vi "update_parameters.vi"(0 "Modify":T1, 9 "Parameters":T2={"Stimulus"={"Type"=enum."Off", "Phase"=0.0, "Amplitude"=[], "Injection point"=enum."Total pose", "Closed loop"=FALSE, "Offset"=[], "Tip -> world"=FALSE, "Frequency"=0.0, "Length"=0.0}, "Goal Filter A"={"Speedup max"=0.0, "Speedup thresh"=0.0, "Speedup nonlin"=0.0, "Filters"=[]}, "Mode controls"={"Hold"=FALSE, "Cancellation"=FALSE, "Goal filter"=FALSE, "Trigger"=FALSE}, "Manipulator type"=enum."Current piezo", "Manipulator calibration"={"Tool offsets"=[[0.0, 0.0, 36200.0]], "Handle light calibration"=[], "Base pivots"=[], "Output pivots"=[], "Length center"=0.0, "Workspace height"=[], "Workspace diameter"=[0.0, 0.0, 36200.0], "Stack travel"=400.0, "Saturation pos"=375.0, "Inverse filters"=[], "Strut length"=0.0}, "Network"={"Remote Host"="", "Send Status"=FALSE, "Send Port"=0, "Recv Commands"=FALSE, "Recv Port"=0}, "Goal Filter B"={"Speedup max"=0.0, "Speedup thresh"=0.0, "Speedup nonlin"=0.0, "Filters"=[]}, "Cancellation"={"KP"={"XY"=0.0, "Rxy"=0.0, "Z"=0.0, "Rz"=0.0}, "KI"=0.0, "KD"={"XY"=0.0, "Rxy"=0.0, "Z"=0.0, "Rz"=0.0}, "Max vel"=20.0, "Max acc"=0.001, "Int error limit"=3.0, "RCM gain"=0.0, "Bypass"=FALSE, "Degraded gain"=0.0}, "Transition time"=0.0, "Estimation"={"Link"={"Measure noise"=[], "Process noise"=[], "Alt process noise"=[], "Alt turnoff cycles"=20, "Innovation limit"=[], "Residue threshold"=0.0, "Enable"=FALSE}, "Handle"={"Measure noise"=[], "Process noise"=[], "State limits"=[], "Innovation limit"=[], "Prediction Lookahead"=0.0, "Enable"=FALSE}}} {"Transition time" format="%_3f"; "Cancellation"."Degraded gain" min=0 max=1 step=0.1 format="%#_3p"; "Cancellation"."RCM gain" min=0 max=1 step=0.1 format="%#_3p"; "Cancellation"."KD"."Rz" min=-1 max=1 step=0.01 format="%#_3p"; "Cancellation"."KD"."Rxy" min=-1 max=1 step=0.01 format="%#_3p"; "Cancellation"."KD"."Z" min=-1 max=1 step=0.01 format="%#_3p"; "Cancellation"."KD"."XY" min=-1 max=1 step=0.01 format="%#_3p"; "Cancellation"."KI" min=0 max=1 step=0.01 format="%#_3p"; "Cancellation"."KP"."Rz" min=-1 max=1 step=0.01 format="%#_3p"; "Cancellation"."KP"."Rxy" min=-1 max=1 step=0.01 format="%#_3p"; "Cancellation"."KP"."Z" min=-1 max=1 step=0.01 format="%#_3p"; "Cancellation"."KP"."XY" min=-1 max=1 step=0.01 format="%#_3p"; "Cancellation"."Max acc" format="%#_3p"; "Goal Filter B"."Filters"."V limit range" format="%_3p"; "Goal Filter B"."Filters"."V limit" format="%_3p"; "Goal Filter B"."Filters"."Upper Q" format="%_3f"; "Goal Filter B"."Filters"."Upper Fc" format="%_3p"; "Goal Filter B"."Filters"."Lower Q" format="%_3f"; "Goal Filter B"."Filters"."Scale factor" format="%_3f"; "Goal Filter B"."Filters"."Lower Fc" format="%_3p"; "Goal Filter B"."Speedup nonlin" format="%_3p"; "Goal Filter B"."Speedup thresh" format="%_3p"; "Goal Filter B"."Speedup max" format="%_3p"; "Manipulator calibration"."Strut length" format="%#_4p"; "Manipulator calibration"."Saturation pos" format="%#.1f"; "Manipulator calibration"."Stack travel" format="%#.1f"; "Manipulator calibration"."Length center" format="%#_4p"; "Manipulator calibration"."Output pivots" format="%#_6f"; "Manipulator calibration"."Base pivots" format="%#_6f"; "Manipulator calibration"."Handle light calibration" format="%#.1f"; "Goal Filter A"."Filters"."V limit range" format="%_3p"; "Goal Filter A"."Filters"."V limit" format="%_3p"; "Goal Filter A"."Filters"."Upper Q" format="%_3f"; "Goal Filter A"."Filters"."Upper Fc" format="%_3p"; "Goal Filter A"."Filters"."Lower Q" format="%_3f"; "Goal Filter A"."Filters"."Scale factor" format="%_3f"; "Goal Filter A"."Filters"."Lower Fc" format="%_3p"; "Goal Filter A"."Speedup nonlin" format="%_3p"; "Goal Filter A"."Speedup thresh" format="%_3p"; "Goal Filter A"."Speedup max" format="%_3p"; "Stimulus"."Length" min=0.0 max=100.0 step=100.0 format="%#_4p"; "Stimulus"."Frequency" min=0.0 step=100.0 format="%#_4g"; "Stimulus"."Offset" format="%#_3p"; "Stimulus"."Amplitude" format="%#_3p"; "Stimulus"."Phase" min=-180.0 max=360.0 step=100.0 format="%#.2f"}, 11 "error in":errorcluster) -> (4 "Changed":bool, 15 "error out":errorcluster)   [LabVIEW 2014]
uses:
  Micron params.ctl
  stimulus.ctl
  injection_point.ctl
  filtering/goal_loop_parms.ctl
  mode_conrols.ctl
  manipulator_cal.ctl
  asap/labview/testing/probe_calibration.ctl
  host/network_params.ctl
  cancellation/sq_control_params.ctl
  cancellation/decoupled_gain.ctl
  cancellation/estimation_controls.ctl
  ui_override_opts.ctl
  initialization/micron_globals.vi
panel:
  out "Old param string":string
  # "True if the current  parameters actually changed."
  # "Modify only these parts of the current parameters.  Other parts of the system may be in charge of other parts of the parameters.  See ui_override.vi, which generates this cluster."
  # "Locals:"
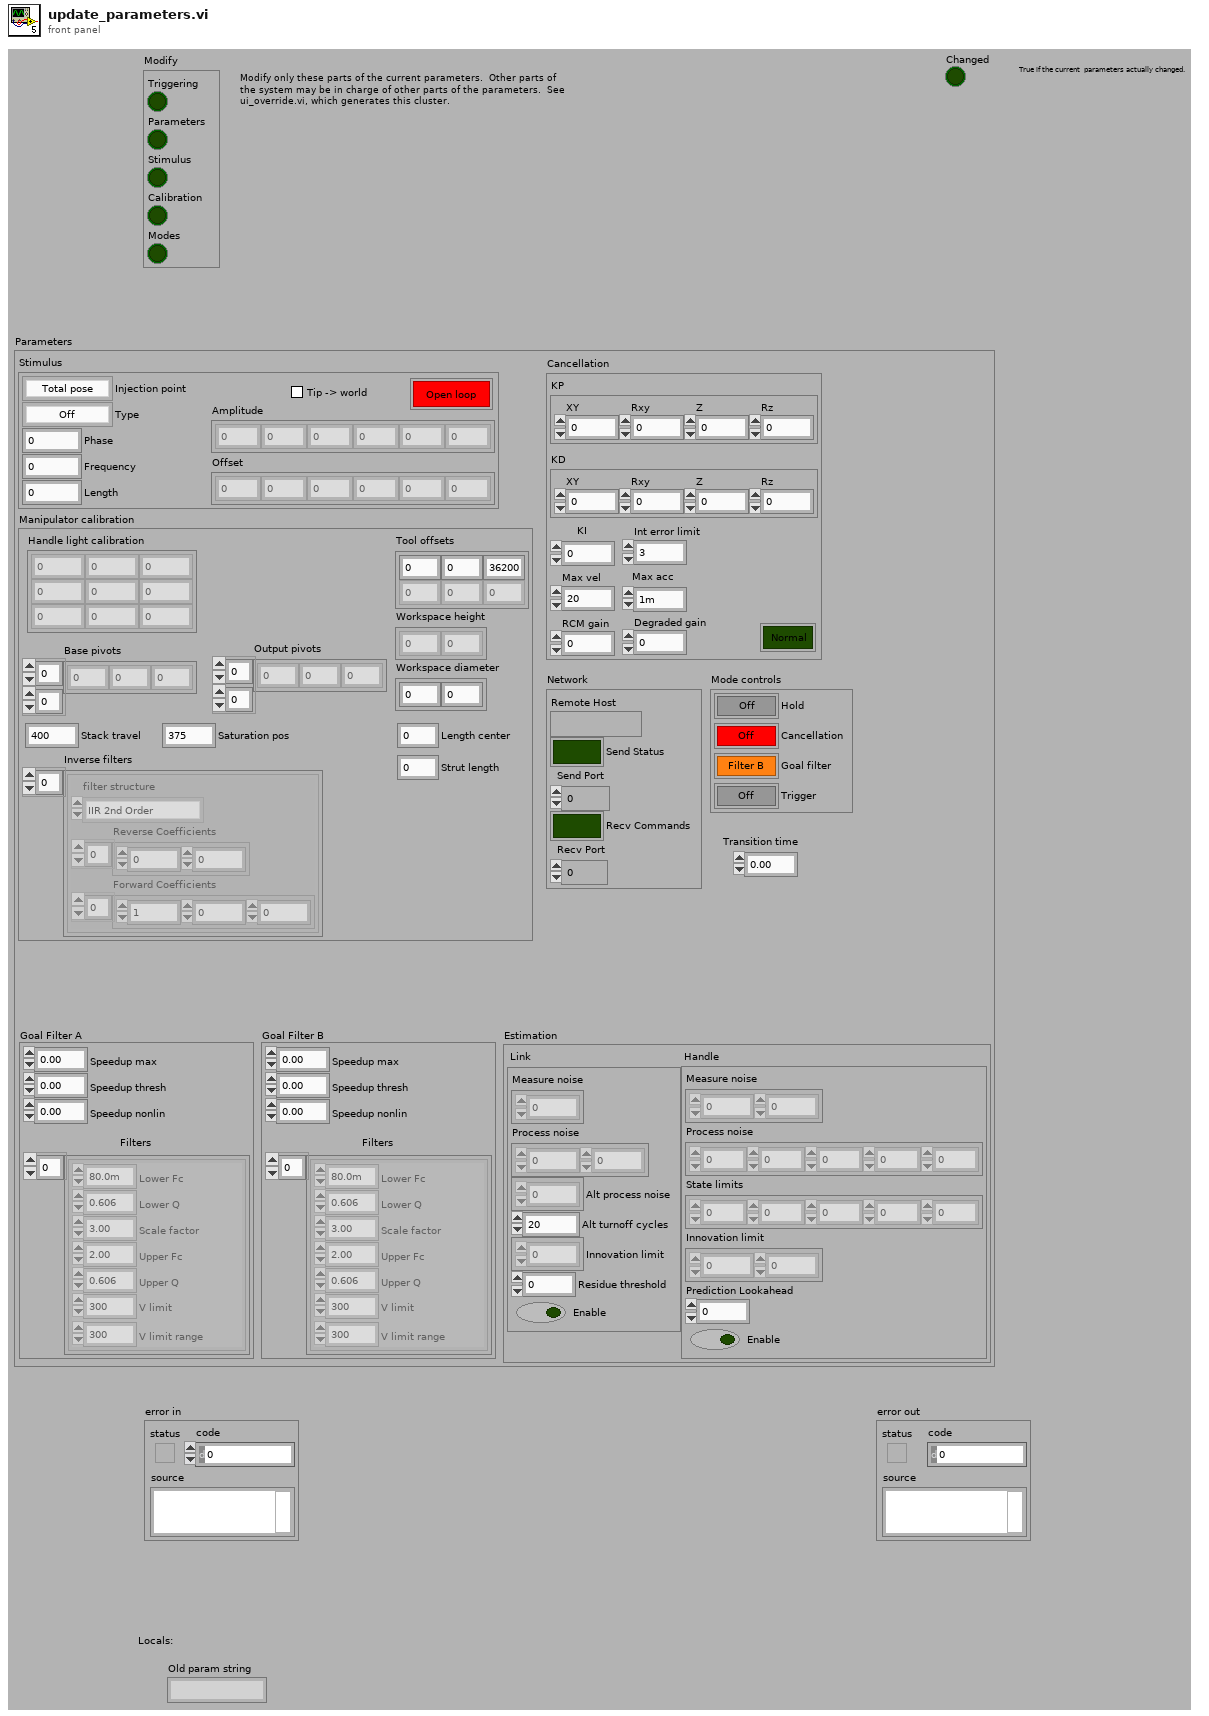
[diagram p1: front panel]
types:
  T1 = typedef "ui_override_opts.ctl" = cluster{"Triggering":bool, "Parameters":bool, "Stimulus":bool, "Calibration":bool, "Modes":bool}
  T2 = typedef "Micron params.ctl" = cluster{"Stimulus":T3, "Goal Filter A":T5, "Mode controls":T6, "Manipulator type":enum16{"Current piezo", "Voltage piezo"}, "Manipulator calibration":T7, "Network":T9, "Goal Filter B":T5, "Cancellation":T10, "Transition time":sgl, "Estimation":T12}
  T3 = typedef "stimulus.ctl" = cluster{"Type":enum16{"Off", "Step", "Sine", "Triangle", "Arbitrary"}, "Phase":dbl, "Amplitude":sgl[], "Injection point":T4, "Closed loop":bool, "Offset":sgl[], "Tip -> world":bool, "Frequency":dbl, "Length":dbl}
  T4 = typedef "injection_point.ctl" = enum16{"Total pose", "V limiter", "Goal ", "Link position", "KF link position", "Inverse kin", "Link goal", "Link error", "Controller", "Output", "Drive", "Light"}
  T5 = typedef "goal_loop_parms.ctl" = cluster{"Speedup max":sgl, "Speedup thresh":sgl, "Speedup nonlin":sgl, "Filters":cluster{"Lower Fc":sgl, "Lower Q":sgl, "Scale factor":sgl, "Upper Fc":sgl, "Upper Q":sgl, "V limit":sgl, "V limit range":sgl}[]}
  T6 = typedef "mode_conrols.ctl" = cluster{"Hold":bool, "Cancellation":bool, "Goal filter":bool, "Trigger":bool}
  T7 = typedef "manipulator_cal.ctl" = cluster{"Tool offsets":sgl[][], "Handle light calibration":T8, "Base pivots":sgl[][], "Output pivots":sgl[][], "Length center":sgl, "Workspace height":sgl[], "Workspace diameter":sgl[], "Stack travel":sgl, "Saturation pos":sgl, "Inverse filters":cluster{"filter structure":enum32{"IIR 2nd Order", "IIR 4th Order"}, "Reverse Coefficients":dbl[], "Forward Coefficients":dbl[]}[], "Strut length":sgl}
  T8 = typedef "probe_calibration.ctl" = sgl[][]
  T9 = typedef "network_params.ctl" = cluster{"Remote Host":string, "Send Status":bool, "Send Port":u16, "Recv Commands":bool, "Recv Port":u16}
  T10 = typedef "sq_control_params.ctl" = cluster{"KP":T11, "KI":sgl, "KD":T11, "Max vel":sgl, "Max acc":sgl, "Int error limit":sgl, "RCM gain":sgl, "Bypass":bool, "Degraded gain":sgl}
  T11 = typedef "decoupled_gain.ctl" = cluster{"XY":sgl, "Rxy":sgl, "Z":sgl, "Rz":sgl}
  T12 = typedef "estimation_controls.ctl" = cluster{"Link":cluster{"Measure noise":dbl[], "Process noise":dbl[], "Alt process noise":dbl[], "Alt turnoff cycles":i32, "Innovation limit":dbl[], "Residue threshold":dbl, "Enable":bool}, "Handle":cluster{"Measure noise":dbl[], "Process noise":dbl[], "State limits":dbl[], "Innovation limit":dbl[], "Prediction Lookahead":sgl, "Enable":bool}}
  T13 = enum16{"Off", "Step", "Sine", "Triangle", "Arbitrary"}
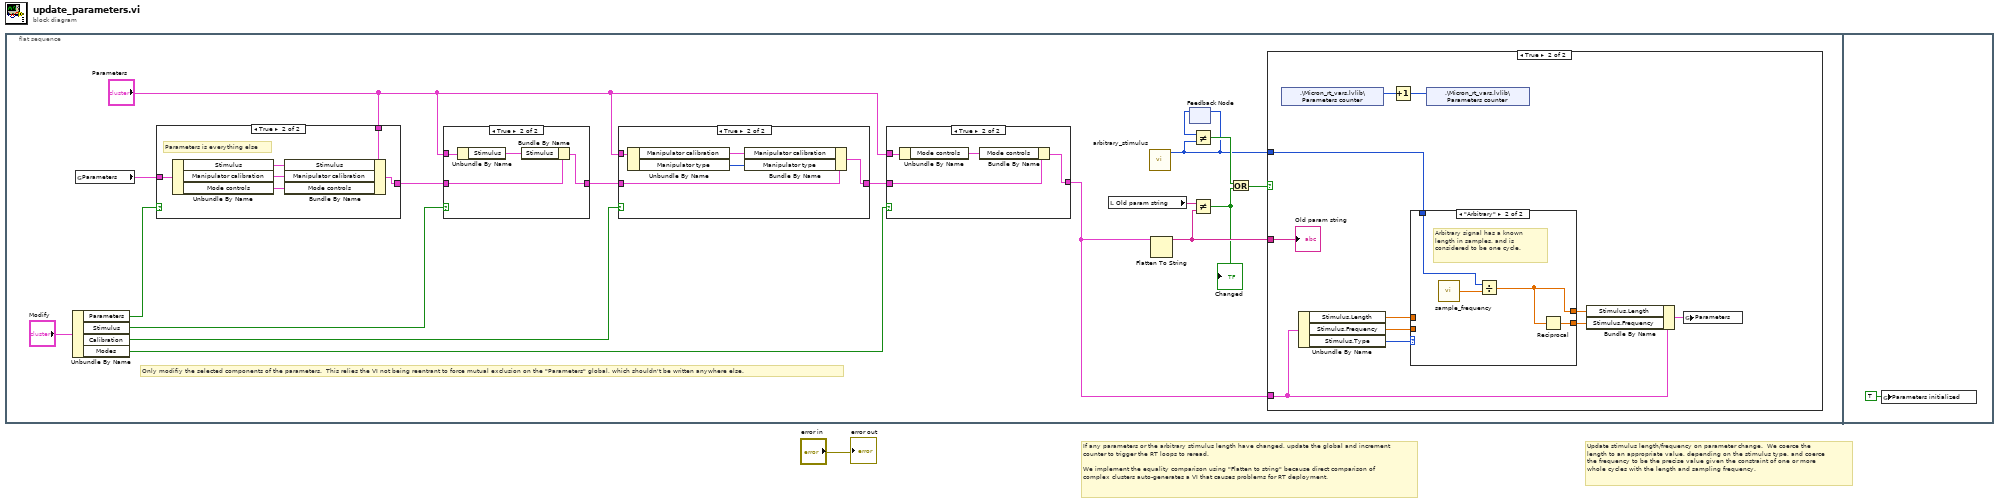
[diagram p0: block diagram]
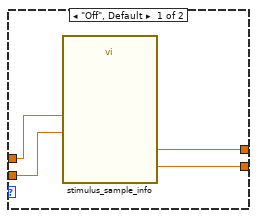
[diagram p7: hidden frame]
diagram:
  # "Update stimulus length/frequency on parameter change.  We coerce the  length to an appropriate value, depending on the stimulus type, and coerce the frequency to be the precise value given the constraint of one or more whole cycles with the length and sampling frequency."
  # "If any parameters or the arbitrary stimulus length have changed, update the global and increment counter to trigger the RT loops to reread.\n\nWe implement the equality comparison using \"Flatten to string\" because direct comparison of complex clusters auto-generates a VI that causes problems for RT deployment."
  n1 = flat-sequence {
    frame #0 {
      # "Only modifiy the selected components of the parameters.  This relies the VI not being reentrant to force mutual exclusion on the \"Parameters\" global, which shouldn't be written anywhere else."
      n2 = Unbundle By Name("Modify") -> ("Parameters"=w6:bool, "Stimulus"=w11:bool, "Calibration"=w10:bool, "Modes"=w7:bool)
      n3 = global read "micron_globals.vi" "Parameters"() -> (w5:T2)
      n4 = case shown="True" w6 {
        tunnel: w5 -> [w20 w26]
        tunnel: "Parameters" -> [_ w25]
        tunnel: [w20 w21] -> w4
        frame False {
        }
        frame True {
          # "Parameters is everything else"
          n5 = Unbundle By Name(w26) -> ("Stimulus"=w24:T3, "Manipulator calibration"=w23:T7, "Mode controls"=w22:T6)
          n6 = Bundle By Name(cluster=w25, "Stimulus"=w24, "Manipulator calibration"=w23, "Mode controls"=w22) -> (w21:T2)
        }
      }
      n7 = case shown="True" w11 {
        tunnel: "Parameters" -> [_ w42]
        tunnel: w4 -> [w38 w41]
        tunnel: [w38 w39] -> w9
        frame False {
        }
        frame True {
          n8 = Unbundle By Name(w42) -> ("Stimulus"=w40:T3)
          n9 = Bundle By Name(cluster=w41, "Stimulus"=w40) -> (w39:T2)
        }
      }
      n10 = case shown="True" w10 {
        tunnel: "Parameters" -> [_ w37]
        tunnel: w9 -> [w32 w36]
        tunnel: [w32 w34] -> w8
        frame False {
        }
        frame True {
          n11 = Unbundle By Name(w37) -> ("Manipulator calibration"=w35:T7, "Manipulator type"=w33:enum16{"Current piezo", "Voltage piezo"})
          n12 = Bundle By Name(cluster=w36, "Manipulator calibration"=w35, "Manipulator type"=w33) -> (w34:T2)
        }
      }
      n13 = case shown="True" w7 {
        tunnel: "Parameters" -> [_ w31]
        tunnel: w8 -> [w27 w30]
        tunnel: [w27 w28] -> w2
        frame False {
        }
        frame True {
          n14 = Unbundle By Name(w31) -> ("Mode controls"=w29:T6)
          n15 = Bundle By Name(cluster=w30, "Mode controls"=w29) -> (w28:T2)
        }
      }
      n16 = local read "Old param string"() -> (w19:string)
      n17 = call "arbitrary_stimulus.vi"() -> ("Length"=w13:i32)  [unwired: 10 in, 1 out]
      n18 = Flatten To String(anything=w2) -> (data string=w18:string)  [unwired: 1 in, 4 out]
      n19 = feedback-in #1(w13) -> ()
      n20 = feedback #1() -> (w17:i32)  [unwired: 1 in]
      n21 = Not Equal?(x=w17, y=w13) -> (x != y?=w15:bool)
      n22 = Not Equal?(x=w19, y=w18) -> (x != y?=w16:bool)
      "Changed" <- w16
      n23 = Or(x=w15, y=w16) -> (x .or. y?=w14:bool)
      n24 = case shown="True" w14 {
        tunnel: w2 -> [_ w46]
        tunnel: w18 -> [_ w51]
        tunnel: w13 -> [_ w45]
        frame False {
        }
        frame True {
          n25 = shared-variable ".\\Micron_rt_vars.lvlib\\Parameters counter"() -> (w52:u32)  [unwired: 2 out]
          n26 = Unbundle By Name(w46) -> ("Stimulus.Length"=w47:dbl, "Stimulus.Frequency"=w48:dbl, "Stimulus.Type"=w49:T13)
          n27 = Increment(x=w52) -> (x+1=w53:u32)
          n28 = case shown="\"Arbitrary\"" w49 {
            tunnel: w48 -> [w56 _]
            tunnel: w47 -> [w57 _]
            tunnel: w45 -> [_ w60]
            tunnel: [w55 w59] -> w44
            tunnel: [w54 w58] -> w43
            frame "Off", Default {
              n29 = call "stimulus_sample_info.vi"("Frequency"=w56, "Length"=w57) -> ("Actual frequency"=w54:dbl, "Actual length"=w55:dbl)  [unwired: 6 in, 2 out]
            }
            frame "Arbitrary" {
              # "Arbitrary signal has a known length in samples, and is considered to be one cycle."
              n30 = call "sample_frequency.vi"() -> ("Sample frequency"=w61:dbl)
              n31 = Divide(x=w60, y=w61) -> (x/y=w59:dbl)
              n32 = Reciprocal(x=w59) -> (1/x=w58:dbl)
            }
          }
          n33 = shared-variable ".\\Micron_rt_vars.lvlib\\Parameters counter"(w53) -> ()  [unwired: 2 out]
          n34 = Bundle By Name(cluster=w46, "Stimulus.Length"=w44, "Stimulus.Frequency"=w43) -> (w50:T2)
          n35 = global write "micron_globals.vi" "Parameters"(w50) -> ()
          "Old param string" <- w51
        }
      }
    }
    frame #1 {
      n36 = global write "micron_globals.vi" "Parameters initialized"(TRUE ("Parameters initialized")) -> ()
    }
  }
  "error out" <- "error in"
